vi "Update Log.vi"(8 "error in (no error)":errorcluster, 10 "Message":string, 11 "UserInterface in":refnum<class "UserInterface.lvclass">) -> (0 "error out":errorcluster, 3 "UserInterface out":refnum<class "UserInterface.lvclass">)   [LabVIEW 2022 SP3, in "UserInterface.lvlib" / "UserInterface.lvclass"]
uses:
  UserInterface.lvclass
  UserInterface.lvclass/UserInterface.ctl
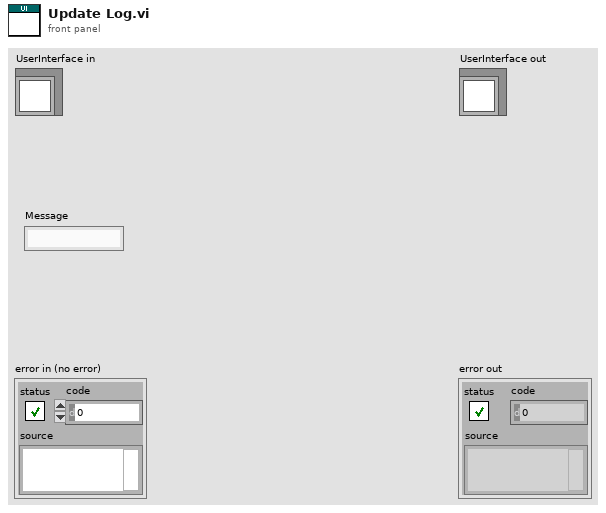
[diagram p1: front panel]
types:
  T1 = cluster{"Image List":refnum<vi>, "ProgressBar":refnum<vi>, "Log":refnum<vi>, "Image Indicator":refnum<vi>}
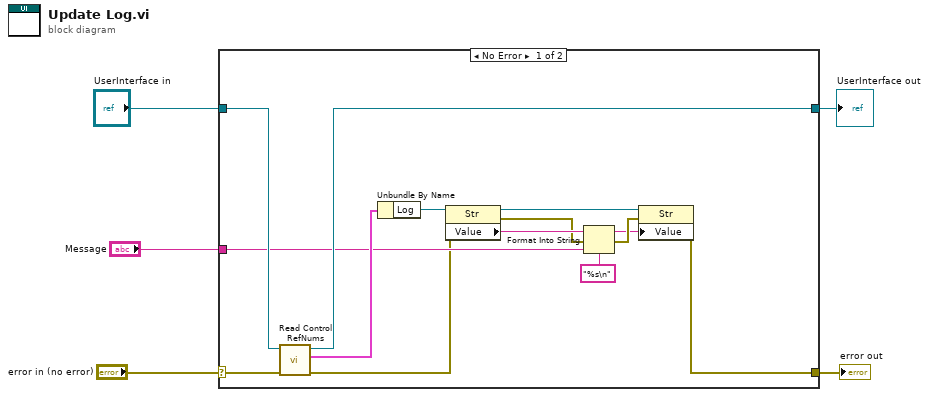
[diagram p0: block diagram]
diagram:
  n1 = case shown="No Error" "error in (no error)" {
    selector: "error in (no error)" -> [w17 w21]
    tunnel: [w6 w21] -> w4
    tunnel: [w18 w20] -> w2
    tunnel: "UserInterface in" -> [w19 w20]
    tunnel: "Message" -> [w11 _]
    frame No Error {
      n2 = call "Read Control RefNums.vi"("error in (no error)"=w17, "UserInterface in"=w19) -> ("error out"=w7:errorcluster, "Control RefNums"=w16:T1, "UserInterface out"=w18:refnum<class "UserInterface.lvclass">)  [unwired: 7 in]
      n3 = Unbundle By Name(w16) -> ("Log"=w15:refnum<vi>)
      n4 = property class="Str"(reference=w15, error in=w7) -> (reference out=w9:refnum<vi>, error out=w12:errorcluster, "Value"=w14:string)
      n5 = Format Into String(format string="%s\n", initial string=w14, error in=w12, w11) -> (resulting string=w8:string, error out=w10:errorcluster)
      n6 = property class="Str"(reference=w9, error in=w10, "Value"=w8) -> (error out=w6:errorcluster)  [unwired: 1 out]
    }
    frame Error {
    }
  }
  "error out" <- w4
  "UserInterface out" <- w2
